vi "TL_define_ROIs_for_display.vi"(3 "XYGraph":refnum<vi>, 4 "error in":errorcluster, 5 "XY positions":dbl[][](array[numeric])) -> (0 "error out":errorcluster, 1 "N Rois":i32, 2 "Mosaic cluster":cluster{dbl[], dbl[]}[](array[cluster]))   [LabVIEW 2015]
uses:
  GLOBAL/Global_CAMERA_TYPE.vi
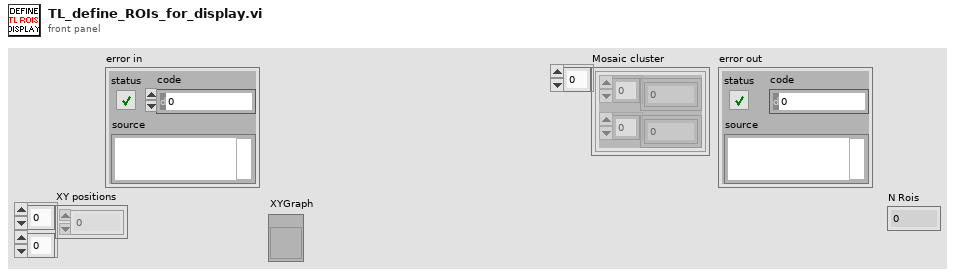
[diagram p1: front panel]
types:
  T1 = typedef "LVRangeTypeDef.ctl" = cluster{"Minimum":dbl, "Maximum":dbl, "Increment":dbl, "Minor Increment":dbl, "Start":dbl}
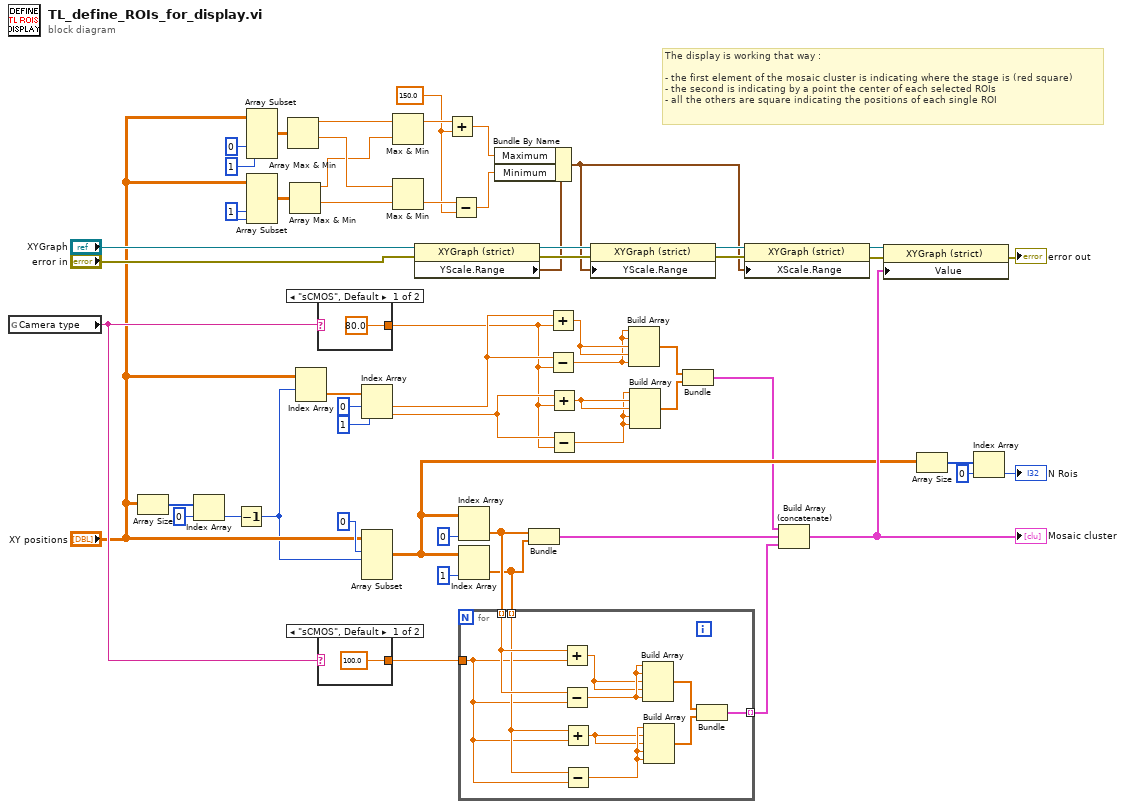
[diagram p0: block diagram]
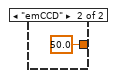
[diagram p2: hidden frame]
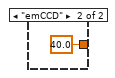
[diagram p3: hidden frame]
diagram:
  w9 = 150.0 ("y")
  w31 = 1 ("index")
  # "The display is working that way :\n\n- the first element of the mosaic cluster is indicating where the stage is (red square)\n- the second is indicating by a point the center of each selected ROIs\n- all the others are square indicating the positions of each single ROI"
  n1 = global read "Global_CAMERA_TYPE.vi" "Camera type"() -> (w6:string)
  n2 = Array Size(array="XY positions") -> (size(s)=w4:i32[])
  n3 = Index Array(array=w4, index=0) -> (element=w2:i32)
  n4 = Decrement(x=w2) -> (x-1=w1:i32)
  n5 = Array Subset(array="XY positions", index (col)=0 ("index"), length (col)=1 ("length")) -> (w28:dbl[][])  [unwired: 2 in]
  n6 = Array Subset(array="XY positions", index (col)=w31, length (col)=w31) -> (w29:dbl[][])  [unwired: 2 in]
  n7 = Array Max & Min(array=w28) -> (max value=w32:dbl, min value=w35:dbl)  [unwired: 2 out]
  n8 = Array Max & Min(array=w29) -> (max value=w33:dbl, min value=w34:dbl)  [unwired: 2 out]
  n9 = Index Array(array="XY positions", index (row)=w1) -> (element=w21:dbl[])  [unwired: 1 in]
  n10 = case shown="\"sCMOS\", Default" w6 {
    tunnel: [80.0 ("y") 40.0 ("y")] -> w8
    frame "sCMOS", Default {
    }
    frame "emCCD" {
    }
  }
  n11 = case shown="\"sCMOS\", Default" w6 {
    tunnel: [100.0 ("y") 50.0 ("y")] -> w7
    frame "sCMOS", Default {
    }
    frame "emCCD" {
    }
  }
  n12 = Index Array(array=w21, index #1=0 ("index"), index #2=1 ("index")) -> (element #1=w13:dbl, element #2=w12:dbl)
  n13 = Array Subset(array="XY positions", index (row)=0 ("index"), length (row)=w1) -> (w22:dbl[][])  [unwired: 2 in]
  n14 = Max & Min(x=w32, y=w33) -> (max(x,y)=w36:dbl)  [unwired: 1 out]
  n15 = Max & Min(x=w35, y=w34) -> (min(x,y)=w37:dbl)  [unwired: 1 out]
  n16 = property class="XYGraph (strict)"(reference="XYGraph", error in="error in") -> (reference out=w54:refnum<vi>, error out=w49:errorcluster, "YScale.Range"=w48:T1)
  n17 = Add(x=w36, y=w9) -> (x+y=w26:dbl)
  n18 = Subtract(x=w37, y=w9) -> (x-y=w25:dbl)
  n19 = Index Array(array=w22, index (col)=0 ("disabled index (col)")) -> (element=w43:dbl[])  [unwired: 1 in]
  n20 = Index Array(array=w22, index (col)=1 ("disabled index (col)")) -> (element=w42:dbl[])  [unwired: 1 in]
  n21 = for {
    tunnel: w43 -> [w67] mode=indexing
    tunnel: w42 -> [w66] mode=indexing
    tunnel: [w63] -> w52 mode=indexing
    tunnel: w7 -> [w62]
    n22 = Add(x=w67, y=w62) -> (x+y=w68:dbl)
    n23 = Subtract(x=w67, y=w62) -> (x-y=w69:dbl)
    n24 = Add(x=w66, y=w62) -> (x+y=w70:dbl)
    n25 = Subtract(x=w66, y=w62) -> (x-y=w71:dbl)
    n26 = Build Array(w69, w69, w68, w68, w69) -> (w65:dbl[])
    n27 = Build Array(w71, w70, w70, w71, w71) -> (w64:dbl[])
    n28 = Bundle(w65, w64) -> (w63:cluster{dbl[], dbl[]})  [unwired: 1 in]
  }
  n29 = Bundle By Name(cluster=w48, "Maximum"=w26, "Minimum"=w25) -> (w24:T1)
  n30 = Bundle(w43, w42) -> (w53:cluster{dbl[], dbl[]})  [unwired: 1 in]
  n31 = Add(x=w13, y=w8) -> (x+y=w16:dbl)
  n32 = Subtract(x=w13, y=w8) -> (x-y=w15:dbl)
  n33 = Add(x=w12, y=w8) -> (x+y=w14:dbl)
  n34 = Subtract(x=w12, y=w8) -> (x-y=w11:dbl)
  n35 = property class="XYGraph (strict)"(reference=w54, error in=w49, "YScale.Range"=w24) -> (reference out=w51:refnum<vi>, error out=w50:errorcluster)
  n36 = Build Array(w15, w15, w16, w16, w15) -> (w17:dbl[])
  n37 = Build Array(w11, w14, w14, w11, w11) -> (w18:dbl[])
  n38 = Bundle(w17, w18) -> (w10:cluster{dbl[], dbl[]})  [unwired: 1 in]
  n39 = property class="XYGraph (strict)"(reference=w51, error in=w50, "XScale.Range"=w24) -> (reference out=w41:refnum<vi>, error out=w40:errorcluster)
  n40 = Build Array (concatenate)(w10, w53, w52) -> (w38:cluster{dbl[], dbl[]}[])
  "Mosaic cluster" <- w38
  n41 = property class="XYGraph (strict)"(reference=w41, error in=w40, "Value"=w38) -> (error out=→"error out":errorcluster)  [unwired: 1 out]
  n42 = Array Size(array=w22) -> (size(s)=w46:i32[])
  n43 = Index Array(array=w46, index=0) -> (element=→"N Rois":i32)
